vi "Create Evaluations.vi"(8 "error in (no error)":errorcluster, 11 "Power Sweep Eval In":refnum<class "Power Sweep.lvclass">) -> (0 "error out":errorcluster, 2 "Evaluations Out":T1[](array[typedef]) {"Low Limit" format="%#_13g"; "SI Scaling" items=["femto"=-15, "pico"=-12, "nano"=-9, "micro"=-6, "milli"=-3, "percent"=-2, ""=0, "kilo"=3, "mega"=6, "giga"=9, "tera"=12]}, 3 "Power Sweep Eval out":refnum<class "Power Sweep.lvclass">)   [LabVIEW 2018, in "SeqAuto Evaluations.lvlib" / "Power Sweep.lvclass"]
uses:
  Power Sweep.lvclass
  C:/Sequence Automation/Plugins/SeqAuto IEvaluation.lvlibp/SeqAuto IEvaluation.lvclass
  Plugins/TestStand API Tools (TSAT).lvlibp/Evaluation Actions/Includes/Controls/TSAT Evaluation.ctl
  Plugins/TestStand API Tools (TSAT).lvlibp/Evaluation Actions/Includes/Controls/TSAT Eval SI Unit Scaling.ctl
  Plugins/TestStand API Tools (TSAT).lvlibp/Evaluation Actions/Includes/Controls/TSAT Evaluation Type.ctl
  Power Sweep.lvclass/Power Sweep.ctl
  Plugins/SeqAuto IEvaluation.lvlibp/Read Measurement Name.vi
  Plugins/TestStand API Tools (TSAT).lvlibp/Evaluation Actions/TSAT Evaluation Actions.lvlib
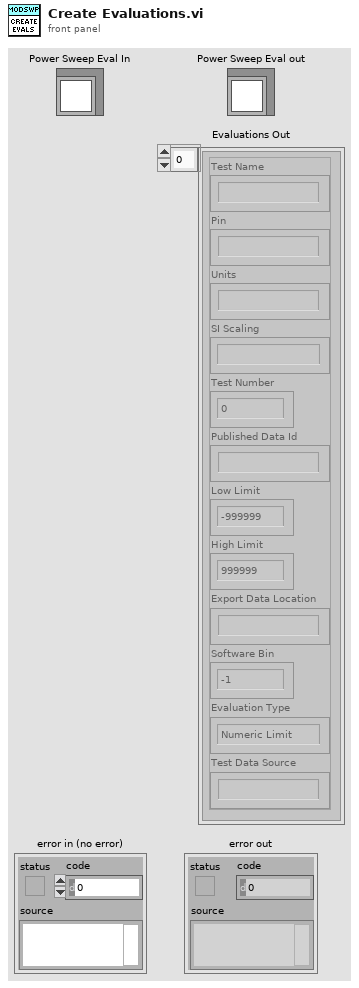
[diagram p1: front panel]
types:
  T1 = typedef "TestStand API Tools (TSAT).lvlibp/TSAT Evaluation Actions.lvlib/TSAT Evaluation.ctl" = cluster{"Test Name":string, "Pin":string, "Units":string, "SI Scaling":T2, "Test Number":i32, "Published Data Id":string, "Low Limit":dbl, "High Limit":dbl, "Export Data Location":string, "Software Bin":i64, "Evaluation Type":T3, "Test Data Source":string}
  T2 = typedef "TestStand API Tools (TSAT).lvlibp/TSAT Evaluation Actions.lvlib/TSAT Eval SI Unit Scaling.ctl" = i16
  T3 = typedef "TestStand API Tools (TSAT).lvlibp/TSAT Evaluation Actions.lvlib/TSAT Evaluation Type.ctl" = enum16{"Numeric Limit", "Pass/Fail", "None"}
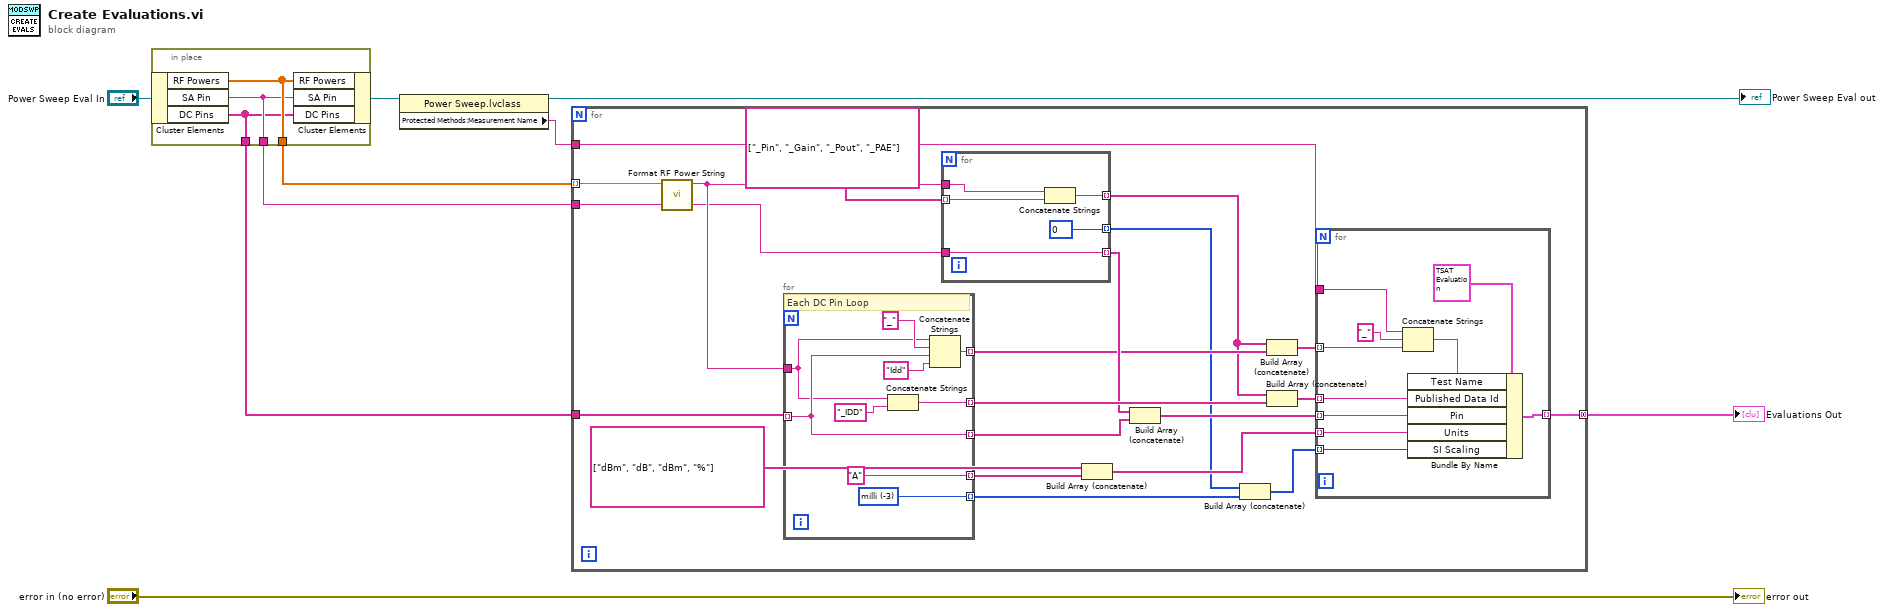
[diagram p0: block diagram]
diagram:
  n1 = in-place {
    in-place-border: [w10] -> w9
    in-place-border: [w11] -> w6
    in-place-border: [w12] -> w7
    n2 = in-place-cluster #1("Power Sweep Eval In") -> ("RF Powers"=w12:dbl[], "SA Pin"=w11:string, "DC Pins"=w10:string[])
    n3 = in-place-cluster #1("RF Powers"=w12, "SA Pin"=w11, "DC Pins"=w10) -> (w1:refnum<class "Power Sweep.lvclass">)
  }
  n4 = property class="Power Sweep.lvclass"(reference=w1) -> (reference out=→"Power Sweep Eval out":refnum<class "Power Sweep.lvclass">, "Protected Methods:Measurement Name"=w8:string)  [unwired: 1 in, 1 out]
  n5 = for {
    tunnel: w9 -> [w18]
    tunnel: w8 -> [w17]
    tunnel: w7 -> [w16] mode=indexing
    tunnel: w6 -> [w14]
    tunnel: [w13] -> w5 mode=concatenating
    n6 = call "Format RF Power String.vi"("x"=w16) -> ("result string"=w15:string)  [unwired: 10 in]
    n7 = for {
      tunnel: w15 -> [w49]
      tunnel: [w56] -> w33 mode=indexing
      tunnel: [w52] -> w30 mode=indexing
      tunnel: w18 -> [w52] mode=indexing
      tunnel: ["A"] -> w27 mode=indexing
      tunnel: [w55] -> w25 mode=indexing
      tunnel: [w54] -> w21 mode=indexing
      w54 = T2 -3 items=["femto"=-15, "pico"=-12, "nano"=-9, "micro"=-6, "milli"=-3, "percent"=-2, ""=0, "kilo"=3, "mega"=6, "giga"=9, "tera"=12] ("SI Scaling")
      # "Each DC Pin Loop"
      n8 = Concatenate Strings(w49, "_IDD" ("string")) -> (w56:string)
      n9 = Concatenate Strings(w49, "_" ("string"), w52, "Idd" ("string")) -> (w55:string)
    }
    n10 = for {
      tunnel: string[] ["_Pin", "_Gain", "_Pout", "_PAE"] -> [w45] mode=indexing
      tunnel: w15 -> [w46]
      tunnel: [w48] -> w24 mode=indexing
      tunnel: [w47] -> w31 mode=indexing
      tunnel: w14 -> [w47]
      tunnel: [w44] -> w22 mode=indexing
      w44 = T2 0 items=["femto"=-15, "pico"=-12, "nano"=-9, "micro"=-6, "milli"=-3, "percent"=-2, ""=0, "kilo"=3, "mega"=6, "giga"=9, "tera"=12] ("SI Scaling")
      n11 = Concatenate Strings(w46, w45) -> (w48:string)
    }
    n12 = Build Array (concatenate)(string[] ["dBm", "dB", "dBm", "%"], w27) -> (w26:string[])
    n13 = Build Array (concatenate)(w31, w30) -> (w29:string[])
    n14 = Build Array (concatenate)(w22, w21) -> (w20:T2[])
    n15 = Build Array (concatenate)(w24, w25) -> (w23:string[])
    n16 = Build Array (concatenate)(w24, w33) -> (w32:string[])
    n17 = for {
      tunnel: w32 -> [w41] mode=indexing
      tunnel: w29 -> [w43] mode=indexing
      tunnel: w26 -> [w42] mode=indexing
      tunnel: w17 -> [w35]
      tunnel: [w39] -> w13 mode=indexing
      tunnel: w23 -> [w38] mode=indexing
      tunnel: w20 -> [w36] mode=indexing
      n18 = Concatenate Strings(w35, "_" ("string"), w38) -> (w37:string)
      n19 = Bundle By Name(cluster=T1 {"Test Name"="", "Pin"="", "Units"="", "SI Scaling"=0, "Test Number"=0, "Published Data Id"="", "Low Limit"=-999999.0, "High Limit"=999999.0, "Export Data Location"="", "Software Bin"=-1, "Evaluation Type"=enum."Numeric Limit", "Test Data Source"=""} ("Evaluation"), "Test Name"=w37, "Published Data Id"=w41, "Pin"=w43, "Units"=w42, "SI Scaling"=w36) -> (w39:T1)
    }
  }
  "Evaluations Out" <- w5
  "error out" <- "error in (no error)"
